vi "Start Triggers Time Core.vi"(2 "tx.trigger select":T4=enum."Immediate", 3 "tx.trigger enable":bool, 4 "tx 0.stream enable":bool, 5 "tx 1.stream enable":bool, 7 "tx.software trigger":bool, 9 "time.resources":T3) -> (15 "tx.start trigger":bool)   [LabVIEW 2015]
uses:
  Host/SubVIs/Start Trigger.ctl
  <instrlib>/niUsrpRio/Time/v1/FPGA/Private/Time Resources.ctl
  <instrlib>/niUsrpRio/Time/v1/FPGA/Private/Future Event Resources.ctl
  <instrlib>/niUsrpRio/Time/v1/FPGA/niUsrpRio Time v1 FPGA.lvlib
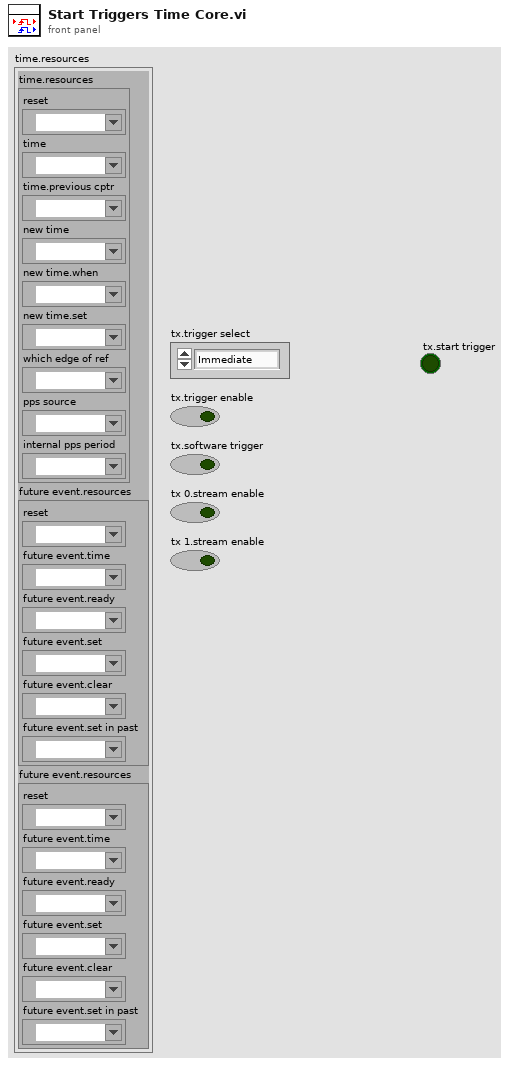
[diagram p1: front panel]
types:
  T1 = typedef "niUsrpRio Time v1 FPGA.lvlib/Time Resources.ctl" = cluster{"reset":refnum<k21>, "time":refnum<k21>, "time.previous cptr":refnum<k21>, "new time":refnum<k21>, "new time.when":refnum<k21>, "new time.set":refnum<k21>, "which edge of ref":refnum<k21>, "pps source":refnum<k21>, "internal pps period":refnum<k21>}
  T2 = typedef "niUsrpRio Time v1 FPGA.lvlib/Future Event Resources.ctl" = cluster{"reset":refnum<k21>, "future event.time":refnum<k21>, "future event.ready":refnum<k21>, "future event.set":refnum<k21>, "future event.clear":refnum<k21>, "future event.set in past":refnum<k21>}
  T3 = cluster{"time.resources":T1, "future event.resources":T2, "future event.resources":T2}
  T4 = typedef "Start Trigger.ctl" = enum8{"Software", "Digital Edge", "Rx Start Trigger", "Tx Start Trigger", "Immediate", "Future Time Event"}
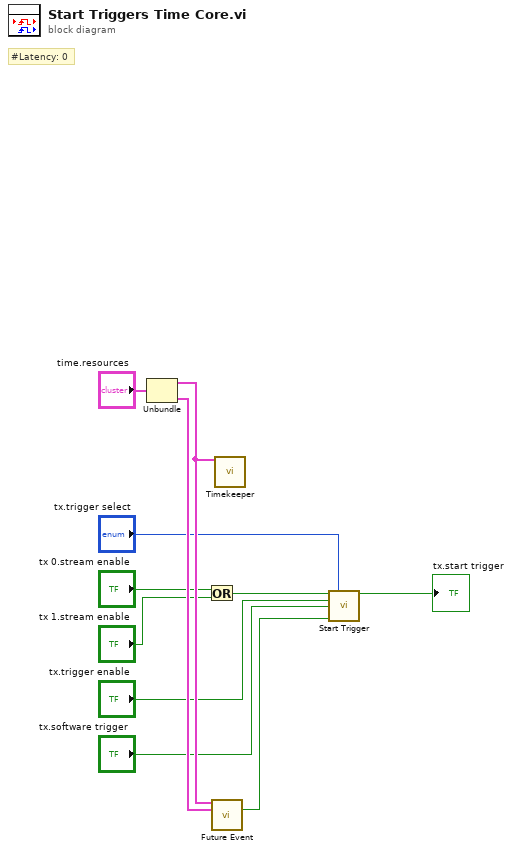
[diagram p0: block diagram]
diagram:
  # "#Latency: 0"
  n1 = Unbundle("time.resources") -> ("time.resources"=w11:T1, "future event.resources"=w10:T2)  [unwired: 1 out]
  n2 = Or(x="tx 0.stream enable", y="tx 1.stream enable") -> (x .or. y?=w4:bool)
  n3 = call <instrlib>:"Future Event.vi"("time.resources"=w11, "future event.resources"=w10) -> ("event.occurred"=w6:bool)  [unwired: 12 in, 1 out]
  n4 = call <instrlib>:"Timekeeper.vi"("time.resources"=w11) -> ()  [unwired: 13 in, 2 out]
  n5 = call "Start Trigger.vi"("stream enable"=w4, "trigger select"="tx.trigger select", "trigger enable"="tx.trigger enable", "software trigger"="tx.software trigger", "event occurred"=w6) -> ("start trigger"=→"tx.start trigger":bool)  [unwired: 10 in]
